vi "Test Template VIs are Ignored.vi"(8 "error in (no error)":errorcluster, 11 "Test Case In":refnum<class "LUnit Test Suite Tests.lvclass">) -> (0 "error out":errorcluster, 3 "Test Case Out":refnum<class "LUnit Test Suite Tests.lvclass">)   [LabVIEW 2020, in "LUnit Test Suite Tests.lvclass"]
uses:
  LUnit Test Suite Tests.lvclass
  LUnit Test Suite Tests.lvclass/LUnit Test Suite Tests.ctl
  Test Doubles/Test Case Test Double Child/Light Test Case Double.lvclass
  <vilib>/Astemes/LUnit/Test Case.lvclass
  source/LUnit Test Suite.lvclass
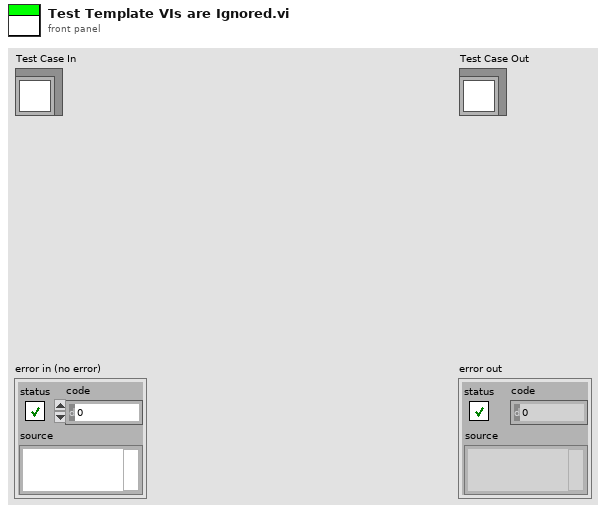
[diagram p1: front panel]
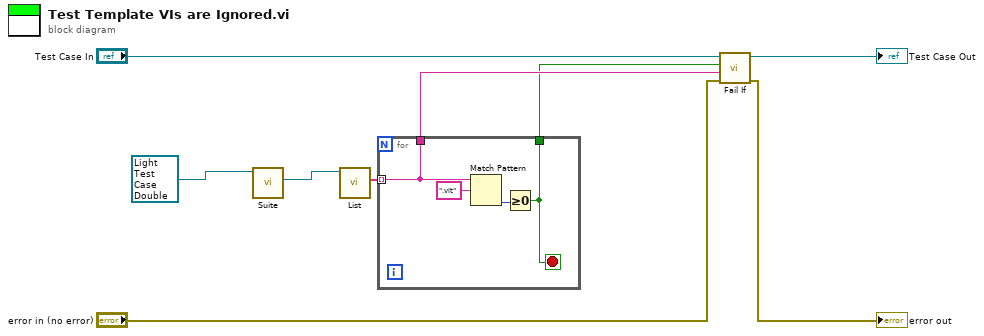
[diagram p0: block diagram]
diagram:
  n1 = call-dynamic "Suite.vi"("LUnit Test Case In"=refnum<class "Light Test Case Double.lvclass"> refnum ("Light Test Case Double.lvclass")) -> ("LUnit Test Suite Out"=w5:refnum<class "LUnit Test Suite.lvclass">)  [unwired: 8 in, 2 out]
  n2 = call "List.vi"("LUnit Test Suite In"=w5) -> ("List of Runnables"=w3:string[])  [unwired: 9 in, 1 out]
  n3 = for {
    tunnel: w3 -> [w11] mode=indexing
    tunnel: [w11] -> w2
    tunnel: [w10] -> w1
    stop <- w10 stop-if-true
    n4 = Match Pattern(string=w11, regular expression=".vit") -> (offset past match=w12:i32)  [unwired: 1 in, 3 out]
    n5 = Greater Or Equal To 0?(x=w12) -> (x >= 0?=w10:bool)
  }
  n6 = call <vilib>:"Fail If.vi"("error in (no error)"="error in (no error)", "Message"=w2, "Fail?"=w1, "LUnit Test Case In"="Test Case In") -> ("error out"=→"error out":errorcluster, "LUnit Test Case Out"=→"Test Case Out":refnum<class "LUnit Test Suite Tests.lvclass">)  [unwired: 6 in]
